vi "Close UniCyRO.vi"(8 "error in (no error)":errorcluster, 11 "UniCyRO_Host in":refnum<class "UniCyRO_Host.lvclass">) -> (0 "error out":errorcluster)   [LabVIEW 2012]
uses:
  UniCyRO_Host.lvclass
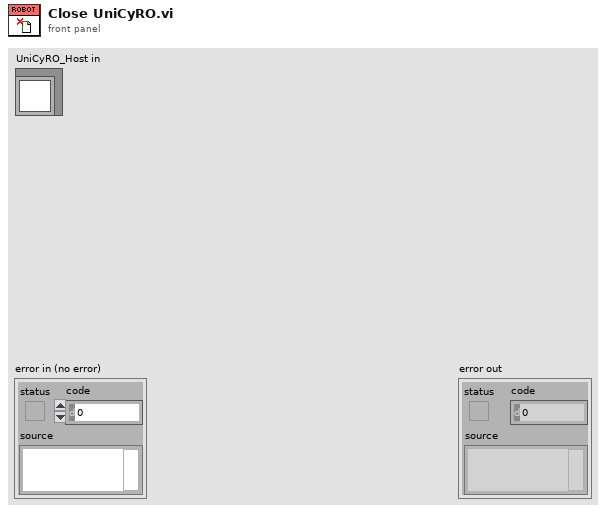
[diagram p1: front panel]
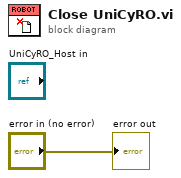
[diagram p0: block diagram]
diagram:
  "error out" <- "error in (no error)"
